vi "Get Intermediate Result.vi"(8 "error in (no error)":errorcluster, 11 "AverageCollector2D in":refnum<class "AverageCollector2D.lvclass">) -> (0 "error out":errorcluster, 2 "AbstractData.lvclass":refnum<class "AbstractData.lvclass">, 3 "AverageCollector2D out":refnum<class "AverageCollector2D.lvclass">)   [LabVIEW 2014, in "AverageCollector2D.lvclass"]
uses:
  AverageCollector2D.lvclass
  Framework/Model/Data/AbstractData/AbstractData.lvclass
  Framework/Collector/AbstractCollector/AbstractCollector.lvclass/AbstractCollector.ctl
  Framework/Model/Data/Data2D/Data2D.lvclass
  Framework/Collector/AbstractCollector/AbstractCollector.lvclass
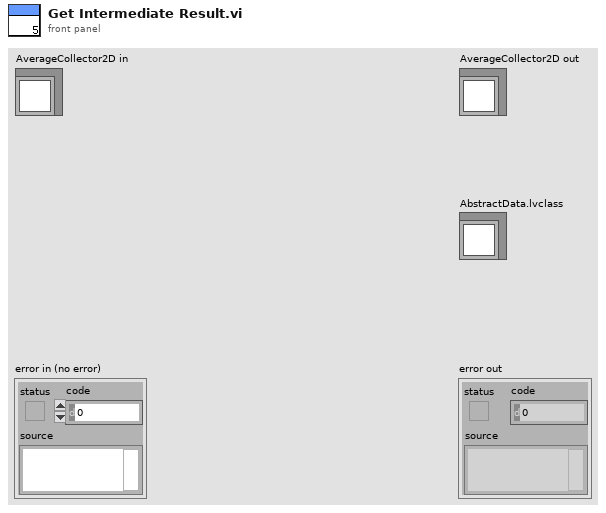
[diagram p1: front panel]
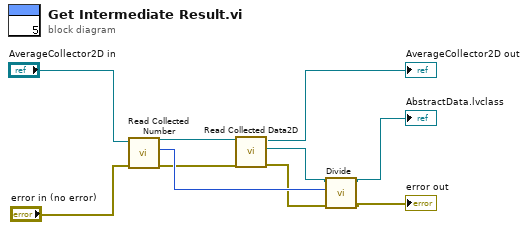
[diagram p0: block diagram]
diagram:
  n1 = call "Read Collected Number.vi"("error in (no error)"="error in (no error)", "AbstractCollector in"="AverageCollector2D in") -> ("error out"=w1:errorcluster, "collected"=w4:u32, "AbstractCollector out"=w8:refnum<class "AverageCollector2D.lvclass">)  [unwired: 7 in]
  n2 = call-dynamic "Read Collected Data2D.vi"("error in (no error)"=w1, "AbstractCollector2D in"=w8) -> ("error out"=w2:errorcluster, "Collected Data"=w5:refnum<class "Data2D.lvclass">, "AbstractCollector2D out"=→"AverageCollector2D out":refnum<class "AverageCollector2D.lvclass">)  [unwired: 7 in]
  n3 = call-dynamic "Divide.vi"("error in (no error)"=w2, "Divider"=w4, "Data2D in"=w5) -> ("error out"=→"error out":errorcluster, "Data2D out"=→"AbstractData.lvclass":refnum<class "Data2D.lvclass">)  [unwired: 7 in]
